vi "PeakHisto.vi"(1 "Data Out":dbl[](array[numeric])) -> (0 "XY Graph":cluster{"Y":dbl[], "Y":dbl[]}[](array[cluster]))   [LabVIEW 2018]
uses:
  Instance           3 17Saved   PeakHisto .vi
  Instance           4 17Saved   PeakHisto .vi
  Instance           2 17Saved   PeakHisto .vi
  <vilib>/Analysis/NI_AALBase.lvlib
panel:
  # "Creates peak amplitude histogram"
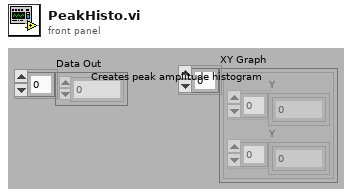
[diagram p1: front panel]
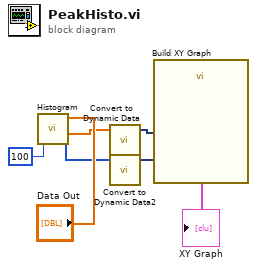
[diagram p0: block diagram]
diagram:
  n1 = call <vilib>:"Histogram.vi"("intervals"=100, "X"="Data Out") -> ("X Values"=w3:dbl[], "Histogram: h(x)"=w5:i32[])  [unwired: 6 in, 2 out]
  n2 = call "Convert to Dynamic Data"("Array"=w3) -> ("Dynamic Data Type"=w4:dynamicdata)  [unwired: 3 in]
  n3 = call "Convert to Dynamic Data2"("Array"=w5) -> ("Dynamic Data Type"=w6:dynamicdata)  [unwired: 3 in]
  n4 = call "Build XY Graph"("Y Input"=w6, "X Input"=w4) -> ("XY Graph"=→"XY Graph":cluster{"Y":dbl[], "Y":dbl[]}[])  [unwired: 8 in, 1 out]
